vi "testAESEncryptDecrypt-CBC-256-AutoIV.vi"(8 "error in (no error)":errorcluster, 11 "TestCase in":refnum<class "TestAES.lvclass">) -> (0 "error out":errorcluster, 3 "TestCase out":refnum<class "TestAES.lvclass">)   [LabVIEW 2021, in "TestAES.lvclass"]
uses:
  TestAES.lvclass
  C:/Program Files (x86)/National Instruments/LabVIEW 2021/vi.lib/addons/_JKI Toolkits/VI Tester/TestCase.llb/TestCase.lvclass
  <vilib>/addons/_JKI Toolkits/VI Tester/TestCase.llb/TestCase.lvclass
  <vilib>/Wiresmith Technology/VITAC (VI Tester Advanced Comparisons)/VITAC.lvlib
  Symmetric Encryption/dotNET Crypto Symmetric Encryption.lvlib
panel:
  out "Encrypted data out":u8[](array[numeric])
  out "IV out":u8[](array[numeric])
  out "Plaintext in (hex)":string="Hello, World!"
  out "Key (hex)":string="01234567890"
  out "Expected plaintext (hex)":string
  out "Actual plaintext out (hex)":string
  out "Expected plaintext":string
  out "Plaintext in":string="Hello, World!"
  out "Actual plaintext out":string
  out "Key":string="01234567890"
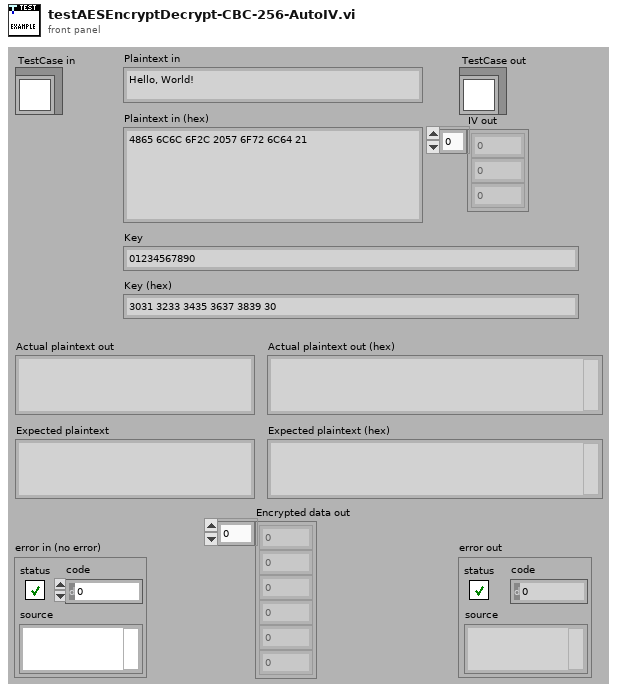
[diagram p1: front panel]
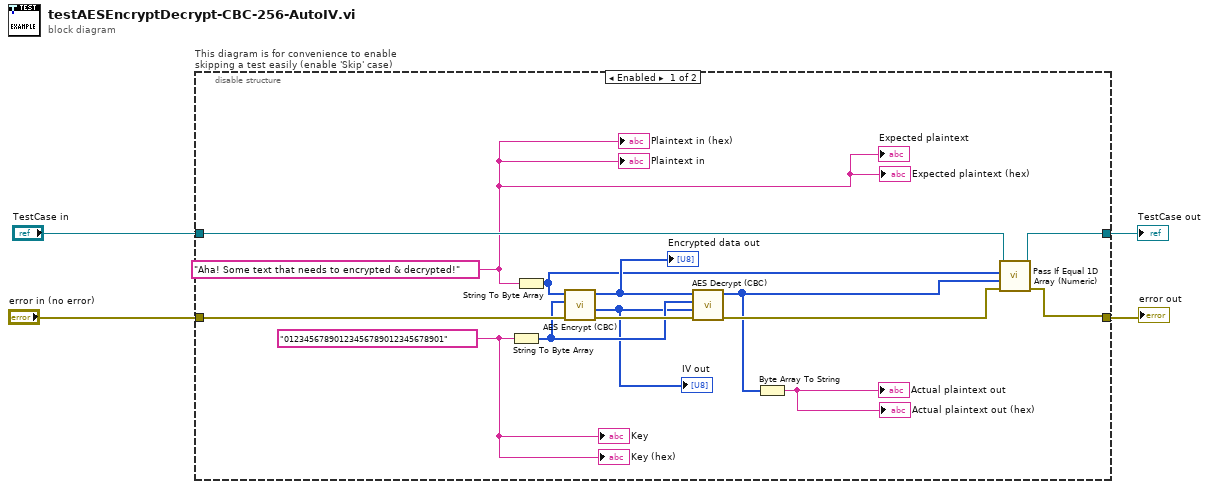
[diagram p0: block diagram]
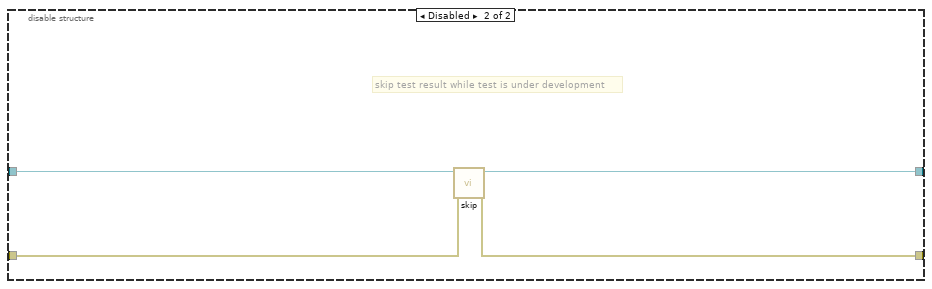
[diagram p2: hidden frame]
diagram:
  n1 = disable-structure "This diagram is for convenience to enable skipping a test easily (enable 'Skip' case)" shown="Enabled" {
    disable-tunnel: "TestCase in" -> [w18 w22]
    disable-tunnel: [w17 w20] -> w1
    disable-tunnel: [w16 w21] -> w3
    disable-tunnel: "error in (no error)" -> [w15 w19]
    frame Enabled {
      w11 = "01234567890123456789012345678901" ("Key")
      w7 = "Aha! Some text that needs to encrypted & decrypted!" ("Plaintext in")
      n2 = String To Byte Array(string=w11) -> (unsigned byte array=w10:u8[])
      n3 = String To Byte Array(string=w7) -> (unsigned byte array=w6:u8[])
      n4 = call "AES Encrypt (CBC).vi"("error in (no error)"=w15, "Key"=w10, "Raw data in"=w6) -> ("error out"=w14:errorcluster, "IV out"=w5:u8[], "Encrypted data out"=w12:u8[])  [unwired: 6 in]
      "IV out" <- w5
      "Encrypted data out" <- w12
      n5 = call "AES Decrypt (CBC).vi"("error in (no error)"=w14, "IV"=w5, "Key"=w10, "Encrypted data in"=w12) -> ("error out"=w13:errorcluster, "Raw data out"=w8:u8[])  [unwired: 6 in]
      n6 = Byte Array To String(unsigned byte array=w8) -> (string=→"Actual plaintext out" →"Actual plaintext out (hex)":string)
      n7 = call <vilib>:"Pass If Equal 1D Array (Numeric).vi"("error in (no error)"=w13, "actual"=w8, "expected"=w6, "TestCase in"=w18) -> ("error out"=w16:errorcluster, "TestCase out"=w17:refnum<class "TestAES.lvclass">)  [unwired: 6 in]
      "Key" <- w11
      "Plaintext in" <- w7
      "Expected plaintext" <- w7
      "Expected plaintext (hex)" <- w7
      "Key (hex)" <- w11
      "Plaintext in (hex)" <- w7
    }
    frame Disabled {
      # "skip test result while test is under development"
      n8 = call <vilib>:"skip.vi"("error in (no error)"=w19, "TestCase in"=w22) -> ("error out"=w21:errorcluster, "TestCase out"=w20:refnum<class "TestAES.lvclass">)  [unwired: 8 in]
    }
  }
  "error out" <- w3
  "TestCase out" <- w1
